vi "Stop SLSC Session Daemon.vi"(8 "error in (no error)":errorcluster, 11 "SLSC Session Handle":T1) -> (0 "error out":errorcluster)   [LabVIEW 2015, in "SLSC Switch.lvlib" / "SLSC Session.lvclass"]
uses:
  SLSC Session/SLSC Session.lvclass
  SLSC Session/Typedefs/Session Handle.ctl
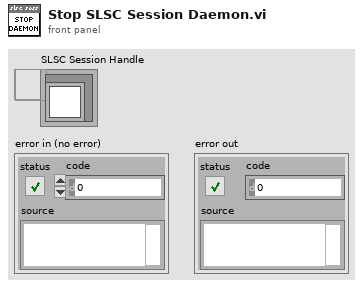
[diagram p1: front panel]
types:
  T1 = typedef "SLSC Switch.lvlib/SLSC Session.lvclass/Session Handle.ctl" = refnum<data-value>
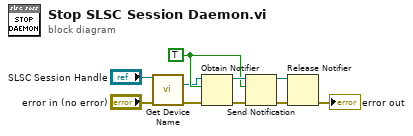
[diagram p0: block diagram]
diagram:
  w5 = TRUE ("notification")
  n1 = call "Get Device Name.vi"("Session Handle in"="SLSC Session Handle", "error in (no error)"="error in (no error)") -> ("device"=w3:refnum<k21>, "error out"=w1:errorcluster)  [unwired: 11 in, 1 out]
  n2 = Obtain Notifier(name (unnamed)=w3, notification data type=w5, error in (no error)=w1) -> (notifier out=w10:refnum<notifier>, error out=w8:errorcluster)  [unwired: 1 in, 1 out]
  n3 = Send Notification(notification=w5, notifier=w10, error in (no error)=w8) -> (notifier out=w9:refnum<notifier>, error out=w7:errorcluster)
  n4 = Release Notifier(notifier=w9, error in (no error)=w7) -> (error out=→"error out":errorcluster)  [unwired: 1 in, 2 out]
